vi "TpControllerMajorOps.vi"() -> (1 "TracepointName":string)   [LabVIEW 2017, in "Controller.lvlib"]
uses:
  <vilib>/addons/InsightCM/Devices/Shared/Common/Controller/Controller.lvlib
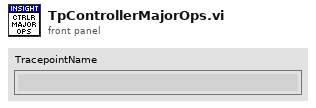
[diagram p1: front panel]
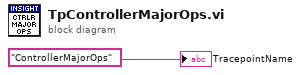
[diagram p0: block diagram]
diagram:
  "TracepointName" <- "ControllerMajorOps" ("ProcessName")
